vi "GT Get Pvt Loop.vi"(7 "pLoop":i32, 8 "error in (no error)":errorcluster caption="错误输入（无错误）", 9 "pLoopCount":i32, 10 "profile":i16, 11 "cardNum":i16) -> (0 "error out":errorcluster caption="错误输出", 1 "pLoopCount out":i32, 3 "function return":i16, 5 "pLoop out":i32)   [LabVIEW 2014, in "gts.lvlib"]
doc: "GT_API GT_GetPvtLoop(short cardNum,short profile,long *pLoopCount,long *pLoop);"
uses:
  gts.lvlib
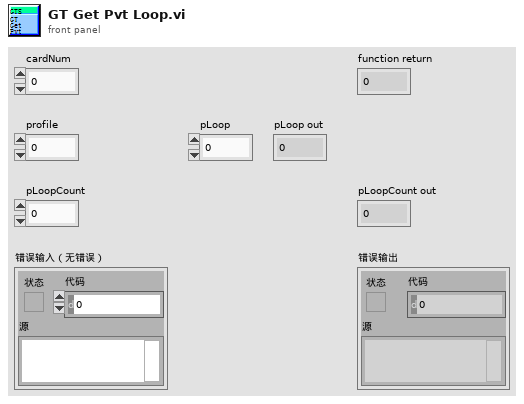
[diagram p1: front panel]
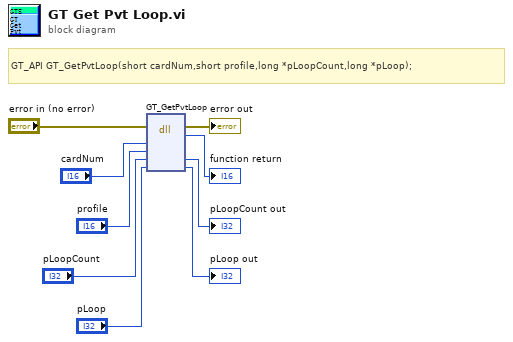
[diagram p0: block diagram]
diagram:
  # "GT_API GT_GetPvtLoop(short cardNum,short profile,long *pLoopCount,long *pLoop);"
  n1 = dll-call lib="PTH2habs D固高科技资料GTS控制卡GTS卡18年上半年资料dllVC32bit\nmulti_cardgts.*" fn="GT_GetPvtLoop"(error in="error in (no error)", "cardNum"="cardNum", "profile"="profile", "pLoopCount"="pLoopCount", "pLoop"="pLoop") -> (error out=→"error out":errorcluster, →"function return":i16, "pLoopCount"=→"pLoopCount out":i32, "pLoop"=→"pLoop out":i32)  [unwired: 4 in, 1 out]
